vi "BarDisplay2Var.vi"(8 "Activation Percentage":dbl, 11 "Target Percentage":dbl) -> ()   [LabVIEW 2016]
panel:
  out "Slide":cluster{dbl, dbl}(slide) scale=0.0..100.0
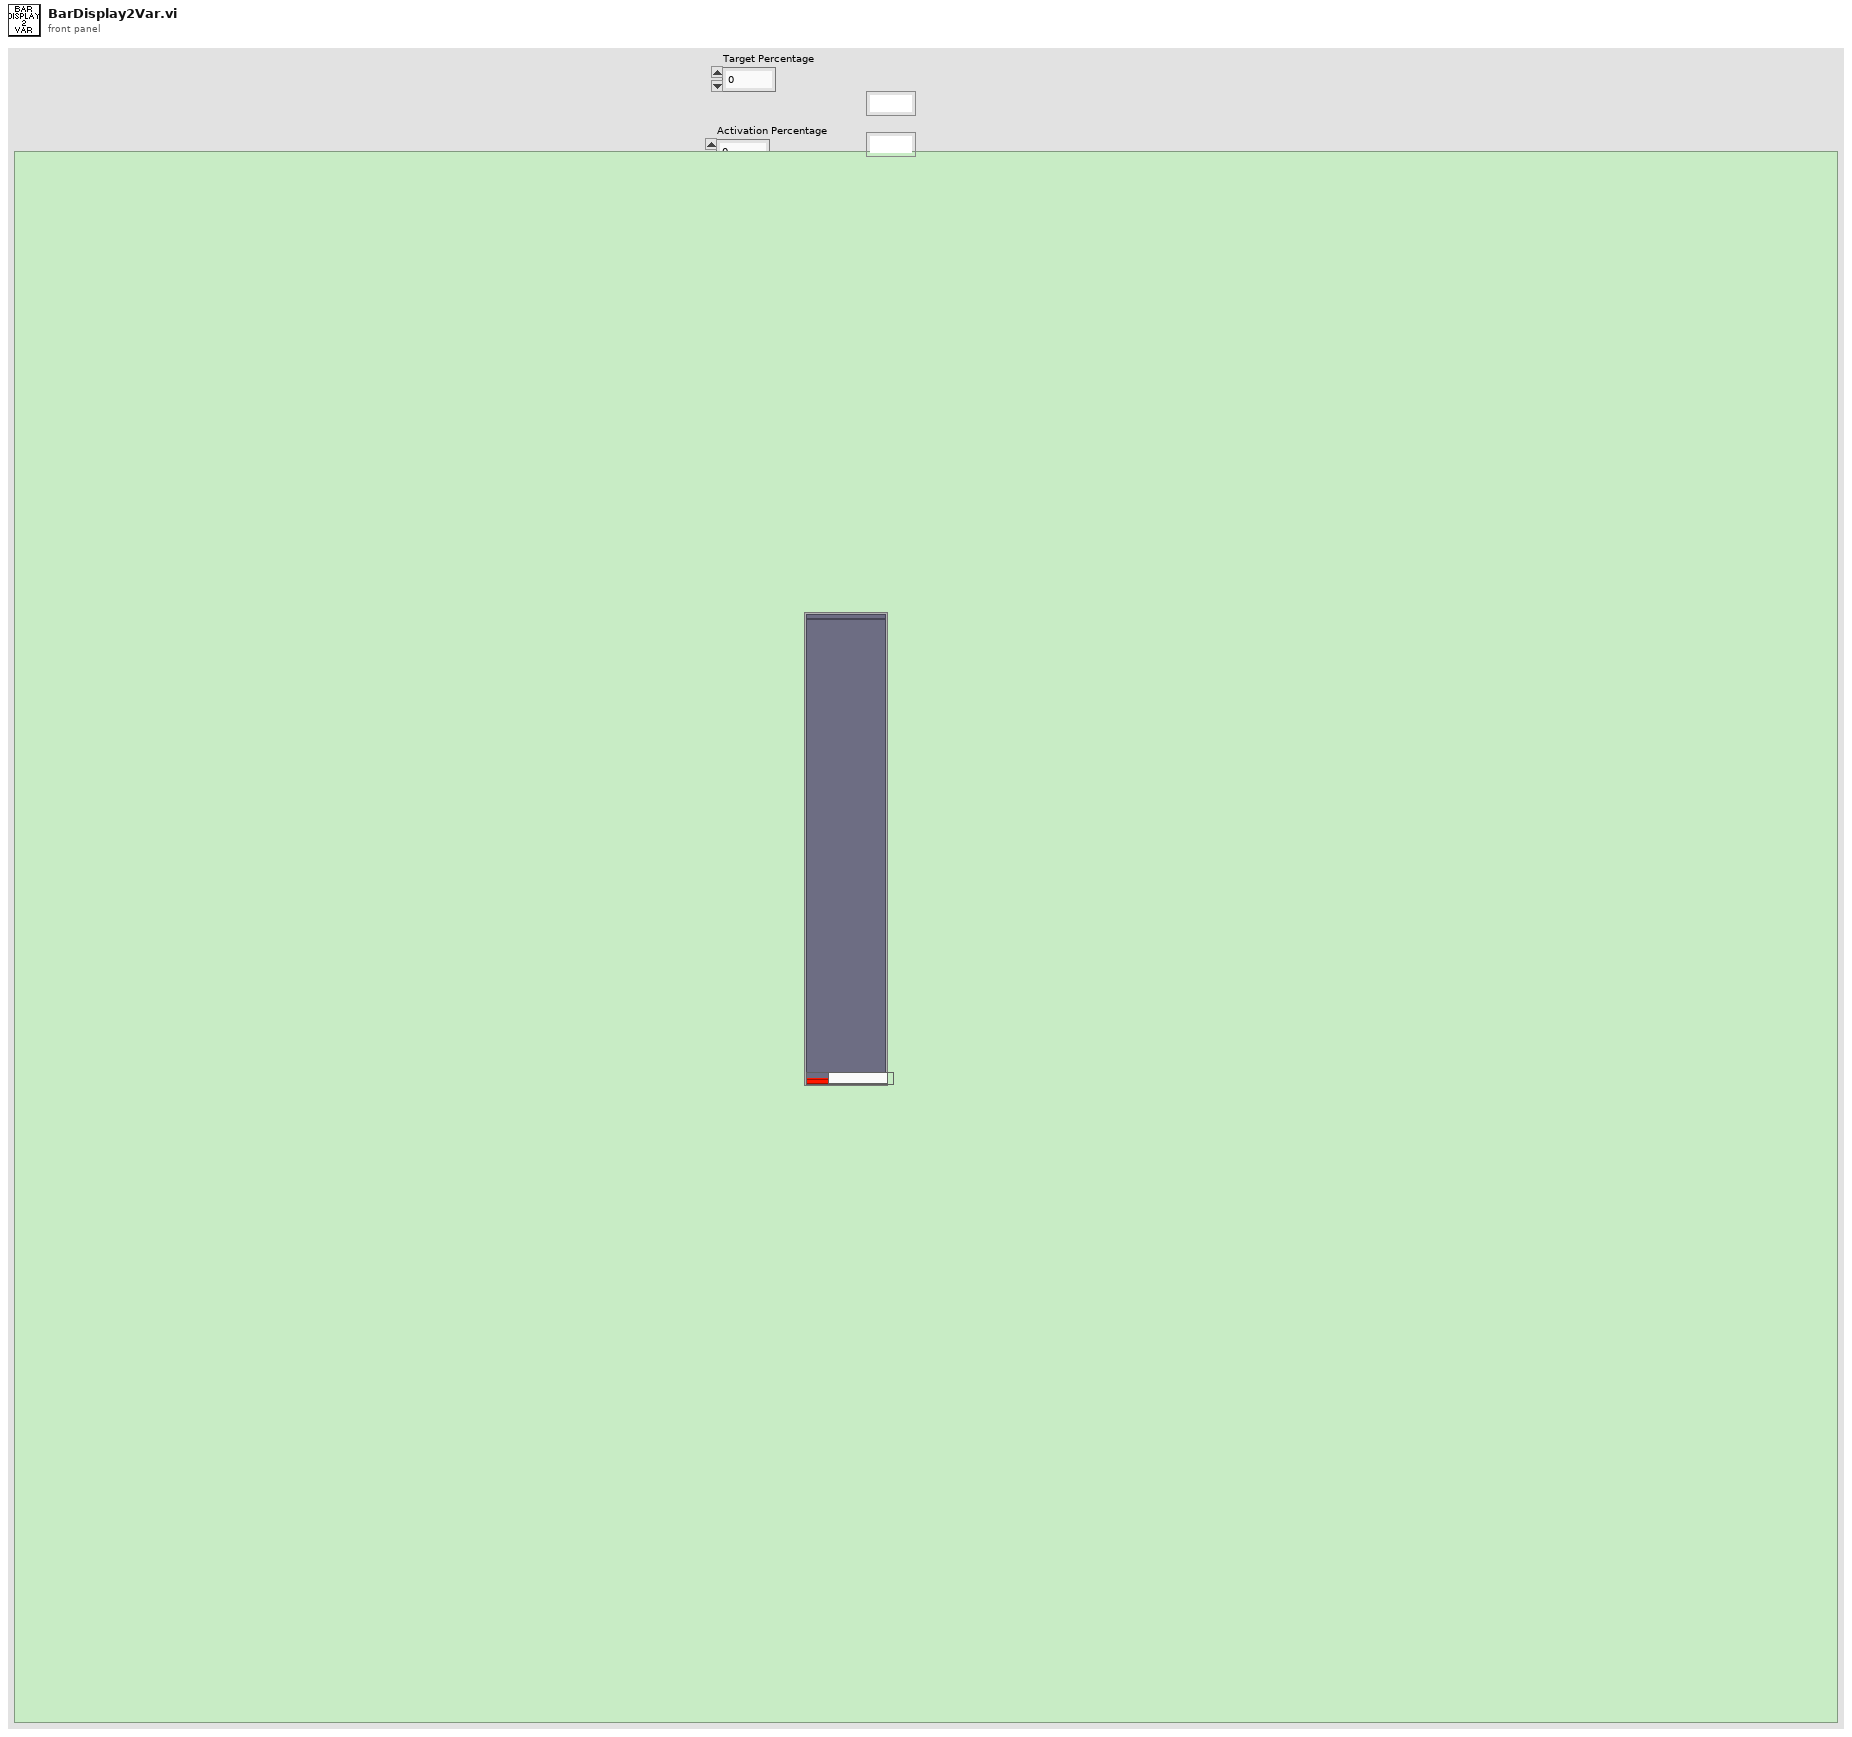
[diagram p1: front panel]
types:
  T1 = cluster{"Target Percentage":dbl, "Activation Percentage":dbl}
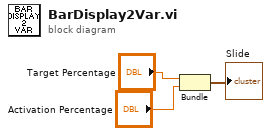
[diagram p0: block diagram]
diagram:
  n1 = Bundle("Target Percentage"="Target Percentage", "Activation Percentage"="Activation Percentage") -> (→"Slide":T1)  [unwired: 1 in]
